vi "GetTraceName.vi"(8 "error in (no error)":errorcluster, 11 "Keysight44xx in":refnum<class "Keysight44xx.lvclass">) -> (0 "error out":errorcluster, 2 "TraceName":string[](array[string]), 3 "Keysight44xx out":refnum<class "Keysight44xx.lvclass">)   [LabVIEW 2018, in "SpecAnPlugins.lvlib" / "Keysight44xx.lvclass"]
doc: "This function returns the specific driver defined trace name that corresponds to the index that the user specifies. If the driver defines a qualified trace name, this property returns the qualified name. If the value that the user passes for the Index parameter is less than one or greater than the value of the Trace Count attribute, the function returns an empty string in the Name parameter and returns the Invalid Value error."
uses:
  Keysight44xx.lvclass
  C:/Users/ico/Documents/Projects/NistPluggableModules/SpecAn/SpecAnPlugins/SpecAnBaseClass/SpecAnBase.lvclass
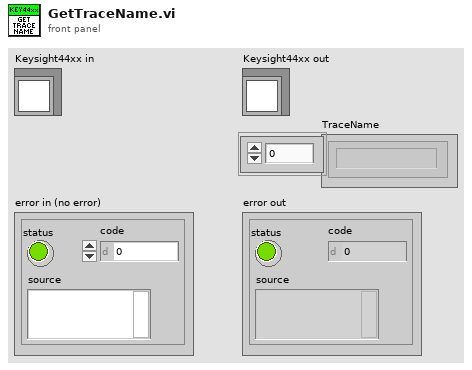
[diagram p1: front panel]
types:
  T1 = typedef "SpecAnPlugins.lvlib/SpecAnBase.lvclass/Trace.ctl" = cluster{"TraceName":string, "TraceSize":i32, "TraceType":i32}[]
  T2 = typedef "SpecAnPlugins.lvlib/SpecAnBase.lvclass/Acquisition.ctl" = cluster{"Handle":string, "Connected":bool, "Enabled":bool, "SweepModeContinuous":bool, "NumberOfSweeps":i32, "DetectorTypeAuto":bool, "DetectorType":i32, "VerticalScale":i32, "MaximumTime(seconds)":dbl}
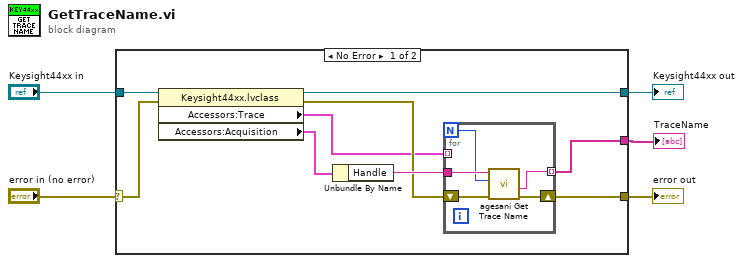
[diagram p0: block diagram]
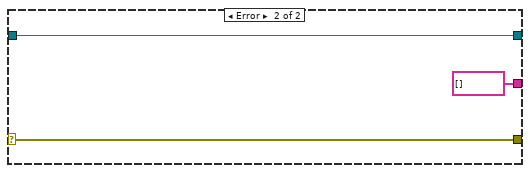
[diagram p2: hidden frame]
diagram:
  n1 = case shown="No Error" "error in (no error)" {
    selector: "error in (no error)" -> [w13 w22]
    tunnel: [w10 w22] -> w4
    tunnel: "Keysight44xx in" -> [w14 w21]
    tunnel: [w12 w21] -> w2
    tunnel: [w8 string[] []] -> w1
    frame No Error {
      n2 = property class="Keysight44xx.lvclass"(reference=w14, error in=w13) -> (reference out=w12:refnum<class "Keysight44xx.lvclass">, error out=w9:errorcluster, "Accessors:Trace"=w7:T1, "Accessors:Acquisition"=w6:T2)
      n3 = Unbundle By Name(w6) -> ("Handle"=w11:string)
      n4 = for {
        N -> [w15]
        tunnel: w11 -> [w19]
        shift-right: [w18] -> w10
        shift-left: w9 -> [w17]
        tunnel: [w16] -> w8 mode=indexing
        tunnel: w7 -> [_] mode=indexing
        n5 = call <instrlib>:"agesani Get Trace Name.vi"("error in (no error)"=w17, "index (1)"=w15, "instrument handle"=w19) -> ("error out"=w18:errorcluster, "name"=w16:string)  [unwired: 6 in, 1 out]
      }
    }
    frame Error {
    }
  }
  "error out" <- w4
  "Keysight44xx out" <- w2
  "TraceName" <- w1
